vi "TrueFalseEnumToBoolean.vi"(10 "error in (no error)":errorcluster, 11 "ChannelOn":enum16{"off", "on"}(ring)) -> (2 "error out":errorcluster, 3 "selection":bool)   [LabVIEW 2020]
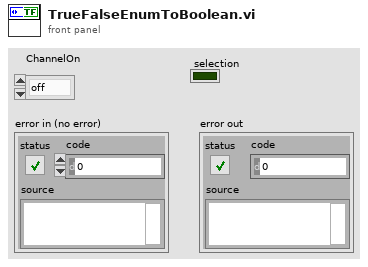
[diagram p1: front panel]
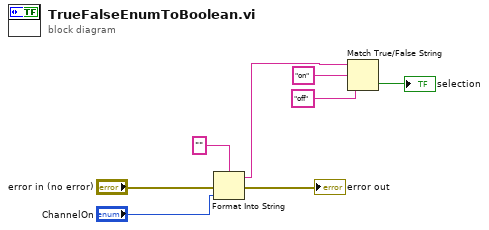
[diagram p0: block diagram]
diagram:
  n1 = Format Into String(format string="", error in="error in (no error)", "ChannelOn") -> (resulting string=w4:string, error out=→"error out":errorcluster)  [unwired: 1 in]
  n2 = Match True/False String(2:"off" ("true string"), 3:"on" ("true string"), 4:w4) -> (0:→"selection":bool)  [unwired: 1 out]
